vi "List.vi"(8 "error in (no error)":errorcluster) -> (0 "error out":errorcluster, 2 "Queues":refnum<queue>[](array[refnum]), 3 "Queue Names":string[](array[string]))   [LabVIEW 2021, in "Queue.lvlib"]
uses:
  Queue.lvlib
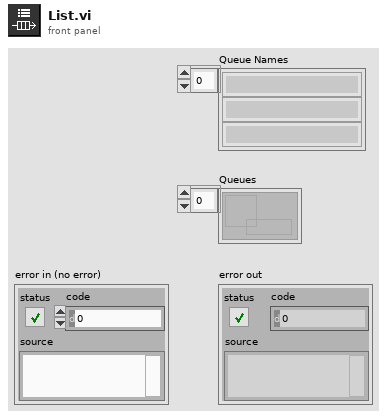
[diagram p1: front panel]
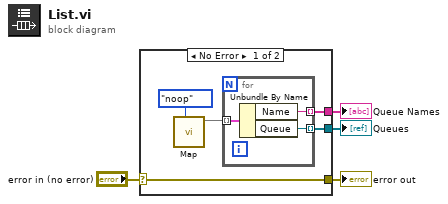
[diagram p0: block diagram]
diagram:
  n1 = case shown="No Error" "error in (no error)" {
    selector: "error in (no error)" -> [w5 w13]
    tunnel: [w7 _] -> w4
    tunnel: [w6 _] -> w3
    tunnel: [w5 w13] -> w2
    frame No Error {
      n2 = call "Map.vi"("Action"=enum8{"noop", "get", "set", "pop"}."noop") -> ("Queue Map"=w8:map{string, refnum<queue>})  [unwired: 8 in, 2 out]
      n3 = for {
        tunnel: w8 -> [w12] mode=indexing
        tunnel: [w11] -> w7 mode=indexing
        tunnel: [w10] -> w6 mode=indexing
        n4 = Unbundle By Name(w12) -> ("Name"=w11:string, "Queue"=w10:refnum<queue>)
      }
    }
    frame Error {
    }
  }
  "error out" <- w2
  "Queue Names" <- w4
  "Queues" <- w3
